vi "Read Key - XML.vi"(8 "error in (no error)":errorcluster, 9 "Key":string, 10 "Section":string, 11 "XML file":path caption="XML file in") -> (0 "error out":errorcluster, 1 "Value Number":i32, 2 "Value String":string, 3 "XML file out":path)   [LabVIEW 2015]
doc: "This vi parses an XML file as if it were an INI file (Section-Key-Value)\n\nInputs \nSection name\nKey Name\n\nOutputs\nKey value"
uses:
  <vilib>/xml/Load XML File.vi
  <vilib>/xml/Close Reference(Node).vi
  <resource>/objmgr/DOMUserDefRef.rc
  <vilib>/xml/NI_XML.lvlib
panel:
  out "XML":string
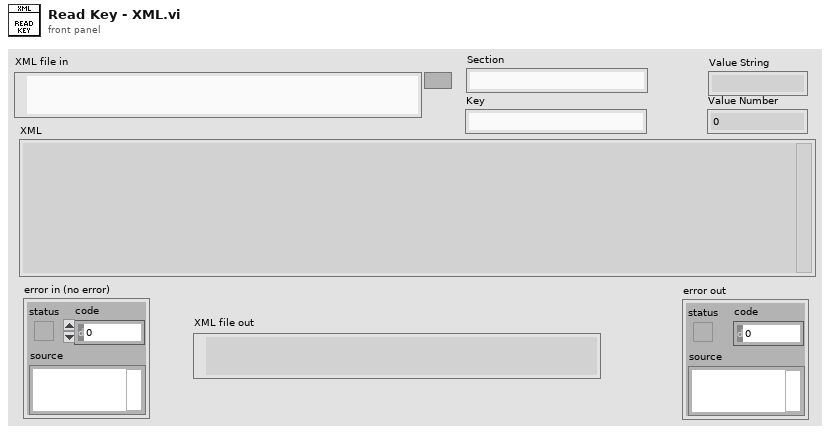
[diagram p1: front panel]
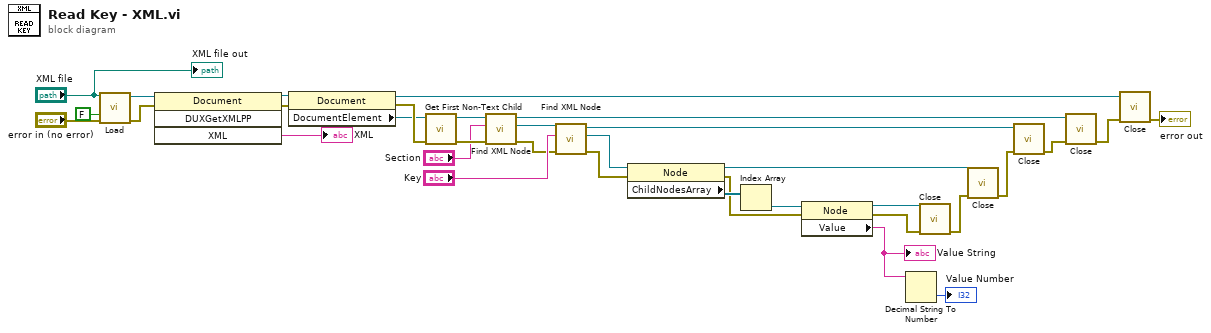
[diagram p0: block diagram]
diagram:
  n1 = call-poly <vilib>:"Load.vi"("path to XML document"="XML file", "load external DTD (True)"=FALSE, "error in (no error)"="error in (no error)") -> ("DOM document out"=w28:refnum<k20>, "error out"=w29:errorcluster)  [unwired: 10 in, 1 out]
  n2 = invoke class="Document" method="DUXGetXMLPP"(reference=w28, error in=w29) -> (reference out=w31:refnum<k20>, error out=w30:errorcluster, "XML"=→"XML":string)  [unwired: 2 in, 1 out]
  n3 = property class="Document"(reference=w31, error in=w30) -> (reference out=w33:refnum<k20>, error out=w34:errorcluster, "DocumentElement"=w23:refnum<k20>)
  n4 = call <vilib>:"Get First Non-Text Child.vi"("error in (no error)"=w34, "node in"=w23) -> ("error out"=w25:errorcluster, "node out"=w24:refnum<k20>)  [unwired: 6 in, 2 out]
  n5 = call "Find XML Node.vi"("error in (no error)"=w25, "Node Name"="Section", "Refnum in"=w24) -> ("error out"=w12:errorcluster, "Node"=w14:refnum<k20>, "Refnum out"=w22:refnum<k20>)  [unwired: 6 in]
  n6 = call "Find XML Node.vi"("error in (no error)"=w12, "Node Name"="Key", "Refnum in"=w14) -> ("error out"=w10:errorcluster, "Node"=w11:refnum<k20>, "Refnum out"=w4:refnum<k20>)  [unwired: 6 in]
  n7 = property class="Node"(reference=w11, error in=w10) -> (reference out=w20:refnum<k20>, error out=w6:errorcluster, "ChildNodesArray"=w19:refnum<k20>[])
  n8 = Index Array(array=w19) -> (element=w18:refnum<k20>)  [unwired: 1 in]
  n9 = property class="Node"(reference=w18, error in=w6) -> (reference out=w9:refnum<k20>, error out=w7:errorcluster, "Value"=w8:string)
  "Value String" <- w8
  n10 = Decimal String To Number(string=w8) -> (number=→"Value Number":i32)  [unwired: 2 in, 1 out]
  n11 = call-poly <vilib>:"Close.vi"("error in (no error)"=w7, "node"=w9) -> ("error out"=w5:errorcluster)  [unwired: 7 in]
  n12 = call-poly <vilib>:"Close.vi"("error in (no error)"=w5, "node"=w20) -> ("error out"=w17:errorcluster)  [unwired: 7 in]
  n13 = call-poly <vilib>:"Close.vi"("error in (no error)"=w17, "node"=w4) -> ("error out"=w16:errorcluster)  [unwired: 7 in]
  n14 = call-poly <vilib>:"Close.vi"("error in (no error)"=w16, "node"=w22) -> ("error out"=w32:errorcluster)  [unwired: 7 in]
  n15 = call-poly <vilib>:"Close.vi"("error in (no error)"=w32, "node"=w33) -> ("error out"=→"error out":errorcluster)  [unwired: 7 in]
  "XML file out" <- "XML file"
